vi "DECODIFICAR ESTADO PIN.vi"(11 "TEXTO":string) -> (2 "number":i32, 3 "concatenated string":string)   [LabVIEW 2019]
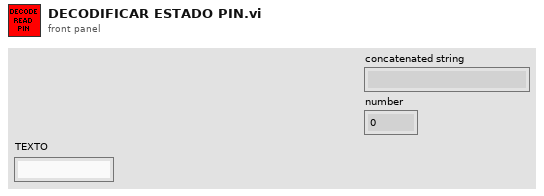
[diagram p1: front panel]
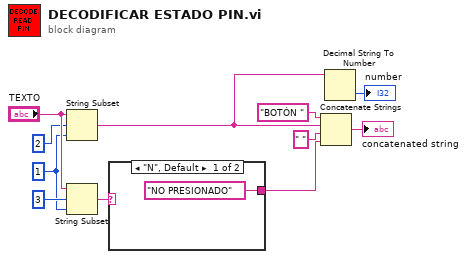
[diagram p0: block diagram]
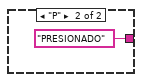
[diagram p2: hidden frame]
diagram:
  w8 = 1 ("length (rest)")
  n1 = String Subset(string="TEXTO", offset (0)=2, length (rest)=w8) -> (substring=w2:string)
  n2 = String Subset(string="TEXTO", offset (0)=3, length (rest)=w8) -> (substring=w7:string)
  n3 = case shown="\"N\", Default" w7 {
    tunnel: ["NO PRESIONADO" "PRESIONADO"] -> w4
    frame "N", Default {
    }
    frame "P" {
    }
  }
  n4 = Concatenate Strings("BOTÓN " ("string"), w2, " " ("string"), w4) -> (→"concatenated string":string)
  n5 = Decimal String To Number(string=w2) -> (number=→"number":i32)  [unwired: 2 in, 1 out]
